vi "GettingStarted.vi"() -> ()   [LabVIEW 2015]
uses:
  <instrlib>/Zurich Instruments LabOne/Public/Configure/ziSetValueDouble.vi
  <instrlib>/Zurich Instruments LabOne/Zurich Instruments LabOne.lvlib
panel:
  out "XY Graph 2":T1(graph)
  out "XY Graph":T1(graph)
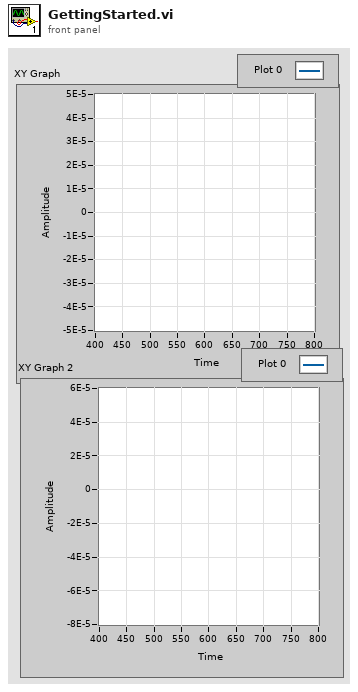
[diagram p1: front panel]
types:
  T1 = cluster{"Output (F,X1,Y1,X2,Y2,...,Vo)":dbl[], "Output (F,X1,Y1,X2,Y2,...,Vo)":dbl[]}
  T2 = typedef "Zurich Instruments LabOne.lvlib/ziTypeHandle.ctl" = cluster{"handleValid":bool, "Conn":u64, "Path Prefix":string, "Handle":u64, "Connected":bool, "Clockbase(s)":dbl}
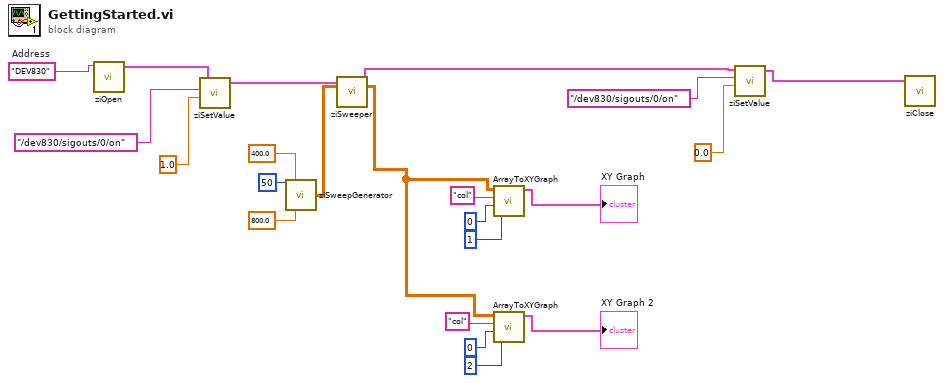
[diagram p0: block diagram]
diagram:
  w22 = "DEV830"  # Address
  n1 = call <instrlib>:"ziOpen.vi"("Address"=w22) -> ("HandleOut"=w21:T2)  [unwired: 3 in, 2 out]
  n2 = call-poly <instrlib>:"ziSetValue.vi"("Value"=1.0, "Path"="/dev830/sigouts/0/on", "Handle In"=w21) -> ("Handle Out"=w18:T2)  [unwired: 2 in, 1 out]
  n3 = call <instrlib>:"ziSweepGenerator.vi"("Steps (#)"=50, "Start (Hz)"=400.0, "Stop (Hz)"=800.0) -> ("Sweep Sequence (F (Hz), BW (Hz), TC(s), Time(s))"=w14:dbl[][])  [unwired: 10 in, 2 out]
  n4 = call <instrlib>:"ziSweeper.vi"("Handle In"=w18, "Sweep Sequence"=w14) -> ("Handle Out"=w3:T2, "Output (F,X1,Y1,X2,Y2,...,Vo)"=w5:dbl[][])  [unwired: 11 in, 1 out]
  n5 = call "ArrayToXYGraph.vi"("input array"=w5, "\"row\" or \"col\""="col", "row or col index for X data"=0 ("index 1"), "row or col index for Y data"=1 ("index 2")) -> ("cluster for XY graph"=→"XY Graph":cluster{"array":dbl[], "array":dbl[]})  [unwired: 5 in]
  n6 = call "ArrayToXYGraph.vi"("input array"=w5, "\"row\" or \"col\""="col", "row or col index for X data"=0 ("index 1"), "row or col index for Y data"=2 ("index 2")) -> ("cluster for XY graph"=→"XY Graph 2":cluster{"array":dbl[], "array":dbl[]})  [unwired: 5 in]
  n7 = call-poly <instrlib>:"ziSetValue.vi"("Value"=0.0, "Path"="/dev830/sigouts/0/on", "Handle In"=w3) -> ("Handle Out"=w2:T2)  [unwired: 2 in, 1 out]
  n8 = call <instrlib>:"ziClose.vi"("Handle In"=w2) -> ()  [unwired: 3 in, 2 out]
